vi "DROPBEAR_Model_Updating_Preprocessing.vi"(8 "error in (no error)":errorcluster, 11 "DROPBEAR_Model_Updating in":refnum<class "DROPBEAR_Model_Updating.lvclass">) -> (0 "error out":errorcluster, 3 "DROPBEAR_Model_Updating out":refnum<class "DROPBEAR_Model_Updating.lvclass">)   [LabVIEW 2021, in "DROPBEAR_Model_Updating.lvclass"]
uses:
  DROPBEAR_Model_Updating.lvclass
  DROPBEAR_Model_Updating.lvclass/DROPBEAR_Model_Updating.ctl
  Read Filter Constants Frequency.vi
  Read Filter Constants Position.vi
  Write Rolling Condition State.vi
  Write Frequency State.vi
  Read Record Time Series Data.vi
  Read Record Moving Window Data.vi
  Read Displacement Measured Nodal .vi
  Read Displacement Measured Meters.vi
  Read Displacement Estimate Nodal.vi
  Read Frequency Measured.vi
  Read Frequency at Estimate.vi
  Read Time Series buffer.vi
  Write Displacement Measured Nodal .vi
  Write Displacement Measured Meters.vi
  Write Displacement Estimate Nodal.vi
  Write Displacement Estimate Meters.vi
  Write Frequency Measured.vi
  Write Frequency at Estimate.vi
  Read Frequency State.vi
  Read Rolling Condition State.vi
  FEA_Model/FEA_Model.lvclass
  MOCKBEAR/MOCKBEAR.lvclass
  Data_Array/Data_Array.lvclass
  Kalman_Filter/Kalman_Filter.lvclass
  Moving_Statistic/Moving_Statistic.lvclass
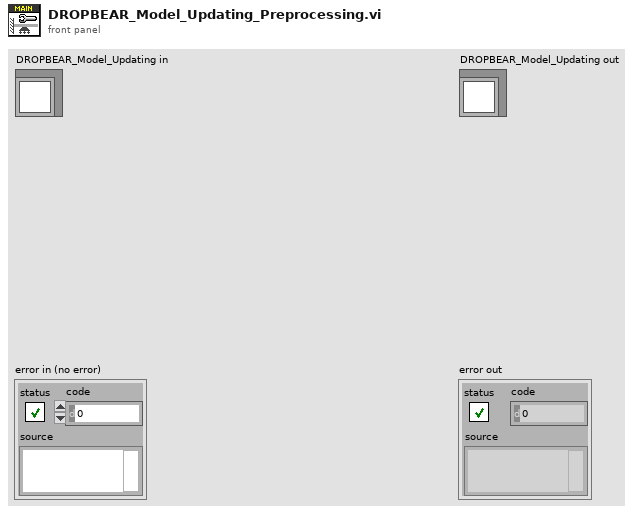
[diagram p1: front panel]
types:
  T1 = cluster{"Modeling Parameters input controls":cluster{"beam_length":dbl, "youngs_modulus":dbl, "torsion_spring":dbl, "beam_height":dbl, "beam_width":dbl, "beam_density":dbl, "number_of_FEA_nodes":i32, "accelerometer_mass":dbl}, "Mockbear input controls":cluster{"Dataset":string, "Resample Method":enum16{"Recorded", "Auto Resample", "Custom Resample"}}, "Simulation Parameters input controls":cluster{"Eigensolver ":enum16{"LabVIEW Cholesky", "LabVIEW General", "LabVIEW Inverse", "LEMP"}, "Models Forcasted":i32, "Max Roller Velocity":dbl, "Max Roller Position Percent":dbl, "Min Roller Position Percent":dbl}, "Program Controls":cluster{"Frequency KF":bool, "Pinned State KF":bool, "FFT Bounding":bool, "Filter Constants Frequency":cluster{"Measurement Variance":dbl, "State Variance":dbl, "Threshold":dbl}, "Filter Constants Position":cluster{"Measurement Variance":dbl, "State Variance":dbl, "Threshold":dbl}, "Moving Window Size":i32, "Time Series buffer":dbl, "Record Time Series Data":bool, "Record Moving Window Data":bool, "Record Online Error Metrics ":bool, "Record Statistics":bool}}
  T2 = cluster{"beam_length":dbl, "youngs_modulus":dbl, "torsion_spring":dbl, "beam_height":dbl, "beam_width":dbl, "beam_density":dbl, "number_of_FEA_nodes":i32, "accelerometer_mass":dbl}
  T3 = cluster{"Dataset":string, "Resample Method":enum16{"Recorded", "Auto Resample", "Custom Resample"}}
  T4 = cluster{"Eigensolver ":enum16{"LabVIEW Cholesky", "LabVIEW General", "LabVIEW Inverse", "LEMP"}, "Models Forcasted":i32, "Max Roller Velocity":dbl, "Max Roller Position Percent":dbl, "Min Roller Position Percent":dbl}
  T5 = cluster{"Measurement Variance":dbl, "State Variance":dbl, "Threshold":dbl}
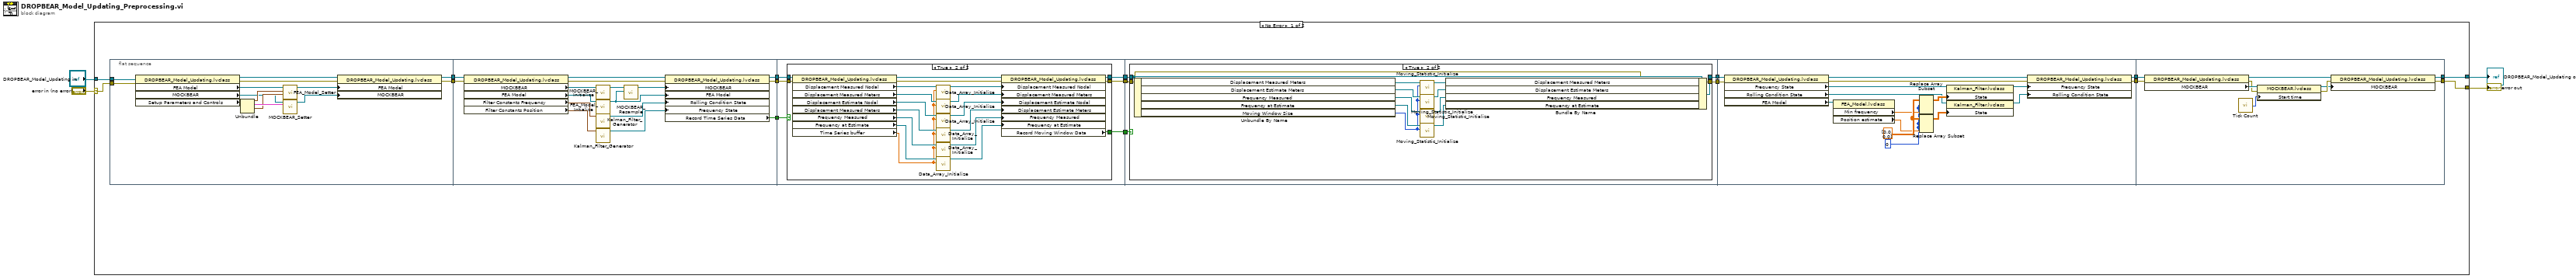
[diagram p0: block diagram]
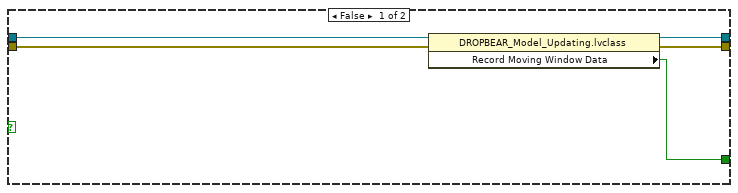
[diagram p2: hidden frame]
diagram:
  n1 = case shown="No Error" "error in (no error)" {
    selector: "error in (no error)" -> [w6 w129]
    tunnel: [w5 w129] -> w3
    tunnel: [w20 w128] -> w1
    tunnel: "DROPBEAR_Model_Updating in" -> [w7 w128]
    frame No Error {
      n2 = flat-sequence {
        tunnel: [w22] -> w9
        tunnel: [w21] -> w8
        tunnel: w7 -> [w24]
        tunnel: w6 -> [w23]
        tunnel: [w39] -> w19
        tunnel: [w38] -> w18
        tunnel: [w37] -> w17
        tunnel: w9 -> [w49]
        tunnel: w8 -> [w35]
        tunnel: [w55] -> w16
        tunnel: w19 -> [w56]
        tunnel: w18 -> [w54]
        tunnel: w17 -> [w53]
        tunnel: [w52] -> w15
        tunnel: [w51] -> w14
        tunnel: w16 -> [w85]
        tunnel: [w86] -> w13
        tunnel: w15 -> [w84]
        tunnel: w14 -> [w83]
        tunnel: [w82] -> w12
        tunnel: [w110] -> w11
        tunnel: w13 -> [w109]
        tunnel: w12 -> [w108]
        tunnel: [w101] -> w10
        tunnel: [w120] -> w20
        tunnel: w11 -> [w127]
        tunnel: w10 -> [w119]
        tunnel: [w118] -> w5
        frame #0 {
          n3 = property class="DROPBEAR_Model_Updating.lvclass"(reference=w24, error in=w23) -> (reference out=w26:refnum<class "DROPBEAR_Model_Updating.lvclass">, error out=w34:errorcluster, "FEA Model"=w25:refnum<class "FEA_Model.lvclass">, "MOCKBEAR"=w30:refnum<class "MOCKBEAR.lvclass">, "Setup Parameters and Controls"=w28:T1)
          n4 = Unbundle(w28) -> ("Modeling Parameters input controls"=w31:T2, "Mockbear input controls"=w33:T3, "Simulation Parameters input controls"=w32:T4)  [unwired: 1 out]
          n5 = call-dynamic "FEA_Model_Setter.vi"("Simulation Parameters input controls"=w32, "Modeling Parameters input controls"=w31, "FEA_Model in"=w25) -> ("FEA_Model out"=w27:refnum<class "FEA_Model.lvclass">)  [unwired: 7 in, 1 out]
          n6 = call-dynamic "MOCKBEAR_Setter.vi"("Mockbear input controls"=w33, "MOCKBEAR in"=w30) -> ("MOCKBEAR out"=w29:refnum<class "MOCKBEAR.lvclass">)  [unwired: 8 in, 1 out]
          n7 = property class="DROPBEAR_Model_Updating.lvclass"(reference=w26, error in=w34, "FEA Model"=w27, "MOCKBEAR"=w29) -> (reference out=w22:refnum<class "DROPBEAR_Model_Updating.lvclass">, error out=w21:errorcluster)
        }
        frame #1 {
          n8 = property class="DROPBEAR_Model_Updating.lvclass"(reference=w49, error in=w35) -> (reference out=w44:refnum<class "DROPBEAR_Model_Updating.lvclass">, error out=w36:errorcluster, "MOCKBEAR"=w48:refnum<class "MOCKBEAR.lvclass">, "FEA Model"=w47:refnum<class "FEA_Model.lvclass">, "Filter Constants Frequency"=w46:T5, "Filter Constants Position"=w45:T5)
          n9 = call-dynamic "MOCKBEAR_Initialize.vi"("MOCKBEAR in"=w48) -> ("MOCKBEAR out"=w50:refnum<class "MOCKBEAR.lvclass">)  [unwired: 9 in, 1 out]
          n10 = call-dynamic "FEA_Model_Intialize.vi"("FEA_Model in"=w47) -> ("FEA_Model out"=w40:refnum<class "FEA_Model.lvclass">)  [unwired: 9 in, 1 out]
          n11 = call "Kalman_Filter_Generator.vi"("Filter Constants"=w46) -> ("Kalman_Filter out"=w43:refnum<class "Kalman_Filter.lvclass">)  [unwired: 9 in, 1 out]
          n12 = call "Kalman_Filter_Generator.vi"("Filter Constants"=w45) -> ("Kalman_Filter out"=w42:refnum<class "Kalman_Filter.lvclass">)  [unwired: 9 in, 1 out]
          n13 = call-dynamic "MOCKBEAR_Resample.vi"("FEA_Model in"=w40, "MOCKBEAR in"=w50) -> ("MOCKBEAR out"=w41:refnum<class "MOCKBEAR.lvclass">)  [unwired: 8 in, 1 out]
          n14 = property class="DROPBEAR_Model_Updating.lvclass"(reference=w44, error in=w36, "MOCKBEAR"=w41, "FEA Model"=w40, "Rolling Condition State"=w43, "Frequency State"=w42) -> (reference out=w39:refnum<class "DROPBEAR_Model_Updating.lvclass">, error out=w38:errorcluster, "Record Time Series Data"=w37:bool)
        }
        frame #2 {
          n15 = case shown="True" w53 {
            tunnel: w56 -> [w61 w81]
            tunnel: [w60 w66] -> w55
            tunnel: w54 -> [w59 w64]
            tunnel: [w58 w63] -> w51
            tunnel: [w57 w62] -> w52
            frame False {
              n16 = property class="DROPBEAR_Model_Updating.lvclass"(reference=w61, error in=w59) -> (reference out=w60:refnum<class "DROPBEAR_Model_Updating.lvclass">, error out=w58:errorcluster, "Record Moving Window Data"=w57:bool)
            }
            frame True {
              n17 = property class="DROPBEAR_Model_Updating.lvclass"(reference=w81, error in=w64) -> (reference out=w67:refnum<class "DROPBEAR_Model_Updating.lvclass">, error out=w65:errorcluster, "Displacement Measured Nodal "=w80:refnum<class "Data_Array.lvclass">, "Displacement Measured Meters"=w79:refnum<class "Data_Array.lvclass">, "Displacement Estimate Nodal"=w78:refnum<class "Data_Array.lvclass">, "Displacement Measured Meters"=w77:refnum<class "Data_Array.lvclass">, "Frequency Measured"=w76:refnum<class "Data_Array.lvclass">, "Frequency at Estimate"=w75:refnum<class "Data_Array.lvclass">, "Time Series buffer"=w74:dbl)
              n18 = call-dynamic "Data_Array_Initialize.vi"("Buffer"=w74, "Data_Array in"=w80) -> ("Data_Array out"=w73:refnum<class "Data_Array.lvclass">)  [unwired: 8 in, 1 out]
              n19 = call-dynamic "Data_Array_Initialize.vi"("Buffer"=w74, "Data_Array in"=w79) -> ("Data_Array out"=w72:refnum<class "Data_Array.lvclass">)  [unwired: 8 in, 1 out]
              n20 = call-dynamic "Data_Array_Initialize.vi"("Buffer"=w74, "Data_Array in"=w78) -> ("Data_Array out"=w71:refnum<class "Data_Array.lvclass">)  [unwired: 8 in, 1 out]
              n21 = call-dynamic "Data_Array_Initialize.vi"("Buffer"=w74, "Data_Array in"=w77) -> ("Data_Array out"=w70:refnum<class "Data_Array.lvclass">)  [unwired: 8 in, 1 out]
              n22 = call-dynamic "Data_Array_Initialize.vi"("Buffer"=w74, "Data_Array in"=w76) -> ("Data_Array out"=w69:refnum<class "Data_Array.lvclass">)  [unwired: 8 in, 1 out]
              n23 = call-dynamic "Data_Array_Initialize.vi"("Buffer"=w74, "Data_Array in"=w75) -> ("Data_Array out"=w68:refnum<class "Data_Array.lvclass">)  [unwired: 8 in, 1 out]
              n24 = property class="DROPBEAR_Model_Updating.lvclass"(reference=w67, error in=w65, "Displacement Measured Nodal "=w73, "Displacement Measured Meters"=w72, "Displacement Estimate Nodal"=w71, "Displacement Estimate Meters"=w70, "Frequency Measured"=w69, "Frequency at Estimate"=w68) -> (reference out=w66:refnum<class "DROPBEAR_Model_Updating.lvclass">, error out=w63:errorcluster, "Record Moving Window Data"=w62:bool)
            }
          }
        }
        frame #3 {
          n25 = case shown="True" w84 {
            tunnel: [w88 w91] -> w86
            tunnel: w85 -> [w88 w90]
            tunnel: w83 -> [w87 w89]
            tunnel: [w87 w89] -> w82
            frame False {
            }
            frame True {
              n26 = Unbundle By Name(w90) -> ("Displacement Measured Meters"=w100:refnum<class "Moving_Statistic.lvclass">, "Displacement Estimate Meters"=w99:refnum<class "Moving_Statistic.lvclass">, "Frequency Measured"=w98:refnum<class "Moving_Statistic.lvclass">, "Frequency at Estimate"=w97:refnum<class "Moving_Statistic.lvclass">, "Moving Window Size"=w96:i32)
              n27 = call-dynamic "Moving_Statistic_Initialize.vi"("Window"=w96, "Moving_Mean in"=w100) -> ("Moving_Mean out"=w95:refnum<class "Moving_Statistic.lvclass">)  [unwired: 8 in, 1 out]
              n28 = call-dynamic "Moving_Statistic_Initialize.vi"("Window"=w96, "Moving_Mean in"=w99) -> ("Moving_Mean out"=w94:refnum<class "Moving_Statistic.lvclass">)  [unwired: 8 in, 1 out]
              n29 = call-dynamic "Moving_Statistic_Initialize.vi"("Window"=w96, "Moving_Mean in"=w98) -> ("Moving_Mean out"=w93:refnum<class "Moving_Statistic.lvclass">)  [unwired: 8 in, 1 out]
              n30 = call-dynamic "Moving_Statistic_Initialize.vi"("Window"=w96, "Moving_Mean in"=w97) -> ("Moving_Mean out"=w92:refnum<class "Moving_Statistic.lvclass">)  [unwired: 8 in, 1 out]
              n31 = Bundle By Name(cluster=w90, "Displacement Measured Meters"=w95, "Displacement Estimate Meters"=w94, "Frequency Measured"=w93, "Frequency at Estimate"=w92) -> (w91:refnum<class "DROPBEAR_Model_Updating.lvclass">)
            }
          }
        }
        frame #4 {
          w111 = 0 ("disabled index (col)")
          w116 = dbl[][] [[0.0], [0.0]] ("array")
          n32 = property class="DROPBEAR_Model_Updating.lvclass"(reference=w109, error in=w108) -> (reference out=w117:refnum<class "DROPBEAR_Model_Updating.lvclass">, error out=w102:errorcluster, "Frequency State"=w107:refnum<class "Kalman_Filter.lvclass">, "Rolling Condition State"=w105:refnum<class "Kalman_Filter.lvclass">, "FEA Model"=w106:refnum<class "FEA_Model.lvclass">)
          n33 = property class="FEA_Model.lvclass"(reference=w106) -> ("Min frequency"=w113:dbl, "Position estimate"=w112:dbl)  [unwired: 1 in, 2 out]
          n34 = Replace Array Subset(array=w116, new element=w113, index (row)=w111, index (col)=w111) -> (w115:dbl[][])
          n35 = Replace Array Subset(array=w116, new element=w112, index (row)=w111, index (col)=w111) -> (w114:dbl[][])
          n36 = property class="Kalman_Filter.lvclass"(reference=w107, "State"=w115) -> (reference out=w103:refnum<class "Kalman_Filter.lvclass">)  [unwired: 1 in, 1 out]
          n37 = property class="Kalman_Filter.lvclass"(reference=w105, "State"=w114) -> (reference out=w104:refnum<class "Kalman_Filter.lvclass">)  [unwired: 1 in, 1 out]
          n38 = property class="DROPBEAR_Model_Updating.lvclass"(reference=w117, error in=w102, "Frequency State"=w103, "Rolling Condition State"=w104) -> (reference out=w110:refnum<class "DROPBEAR_Model_Updating.lvclass">, error out=w101:errorcluster)
        }
        frame #5 {
          n39 = property class="DROPBEAR_Model_Updating.lvclass"(reference=w127, error in=w119) -> (reference out=w121:refnum<class "DROPBEAR_Model_Updating.lvclass">, error out=w124:errorcluster, "MOCKBEAR"=w126:refnum<class "MOCKBEAR.lvclass">)
          n40 = call "Tick Count"() -> ("Tick Count(uSec)"=w125:u32)
          n41 = property class="MOCKBEAR.lvclass"(reference=w126, error in=w124, "Start time"=w125) -> (reference out=w122:refnum<class "MOCKBEAR.lvclass">, error out=w123:errorcluster)
          n42 = property class="DROPBEAR_Model_Updating.lvclass"(reference=w121, error in=w123, "MOCKBEAR"=w122) -> (reference out=w120:refnum<class "DROPBEAR_Model_Updating.lvclass">, error out=w118:errorcluster)
        }
      }
    }
    frame Error {
    }
  }
  "error out" <- w3
  "DROPBEAR_Model_Updating out" <- w1
